vi "myRIO_BRig_RT_dataExp_TPB_max__L.vi"() -> (2 "output_TPB_max__L":i32)   [LabVIEW 2014]
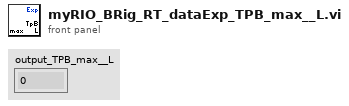
[diagram p1: front panel]
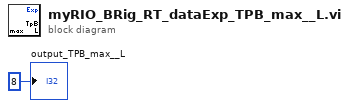
[diagram p0: block diagram]
diagram:
  "output_TPB_max__L" <- 8 ("output_iBlock")
